vi "openSubProcess.vi"(6 "Device IDN":string, 8 "error in (no error)":errorcluster {"code" format="Error %.0f"}, 10 "notifiers":T2, 11 "messageQueues":T3) -> (0 "error out":errorcluster {"code" format="Error %.0f"}, 3 "SubViRefsOut":T1)   [LabVIEW 2017]
doc: "This VI will open and pass messageQueues and Notifier clusters to each subpanel process."
uses:
  Message Queues/messageQueues.ctl
  Message Queues/Message Cluster.ctl
  Notifiers/notifiers.ctl
  Controls/SubViRefs.ctl
  <vilib>/Utility/error.llb/Error Cluster From Error Code.vi
  <vilib>/ErrorRing/Error Ring.xnode
  Message Queues/Message Queue.lvlib
  Notifiers/notifiers.lvlib
panel:
  in  "SubViRefs":T1
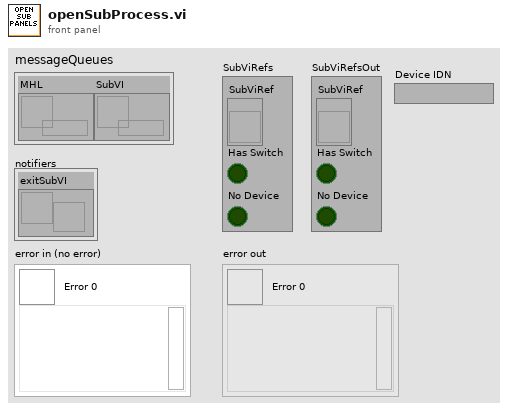
[diagram p1: front panel]
types:
  T1 = typedef "SubViRefs.ctl" = cluster{"SubViRef":refnum<vi>, "Has Switch":bool, "No Device":bool}
  T2 = typedef "notifiers.lvlib/notifiers.ctl" = cluster{"exitSubVI":refnum<notifier>}
  T3 = typedef "Message Queue.lvlib/messageQueues.ctl" = cluster{"MHL":refnum<queue>, "SubVI":refnum<queue>}
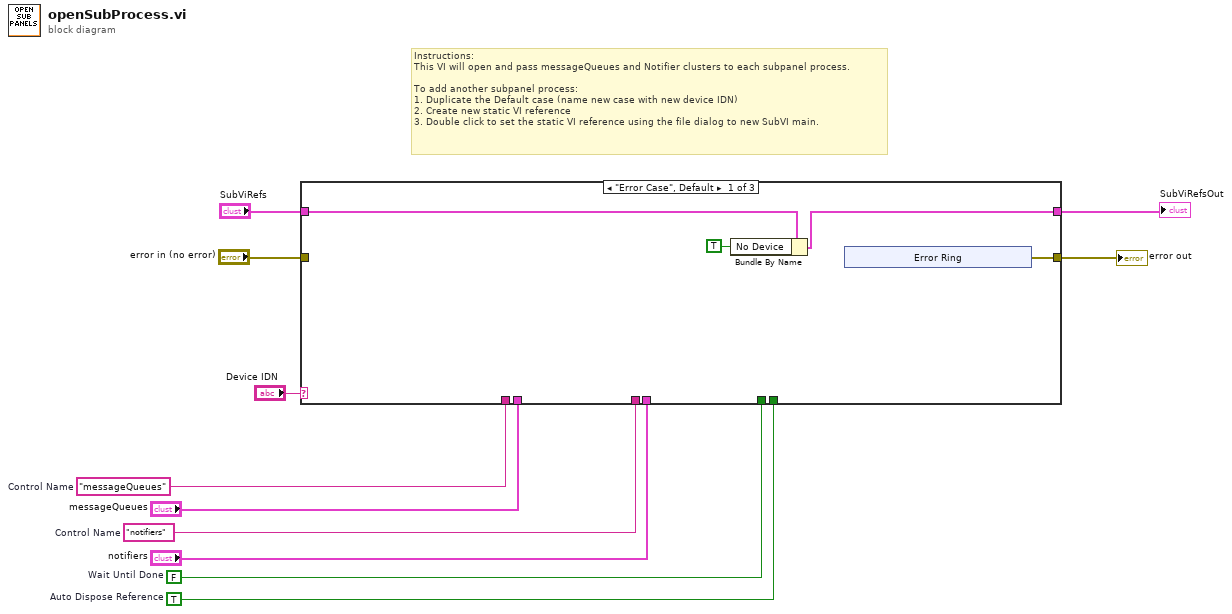
[diagram p0: block diagram]
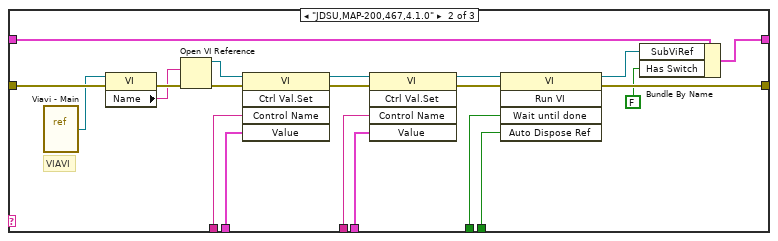
[diagram p2: hidden frame]
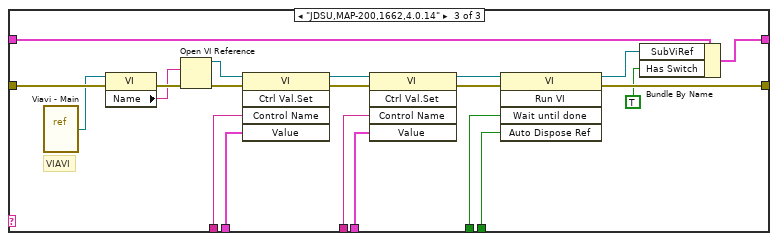
[diagram p3: hidden frame]
diagram:
  w7 = "notifiers"  # Control Name
  w4 = TRUE  # Auto Dispose Reference
  w5 = FALSE  # Wait Until Done
  w9 = "messageQueues"  # Control Name
  # "Instructions:\nThis VI will open and pass messageQueues and Notifier clusters to each subpanel process.\n\nTo add another subpanel process:\n1. Duplicate the Default case (name new case with new device IDN)\n2. Create new static VI reference\n3. Double click to set the static VI reference using the file dialog to new SubVI main."
  n1 = case shown="\"Error Case\", Default" "Device IDN" {
    tunnel: "error in (no error)" -> [_ w33 w54]
    tunnel: "SubViRefs" -> [w14 w31 w52]
    tunnel: [w13 w30 w51] -> w2
    tunnel: [w15 w29 w50] -> w10
    tunnel: w9 -> [_ w28 w49]
    tunnel: "messageQueues" -> [_ w27 w48]
    tunnel: w7 -> [_ w26 w47]
    tunnel: "notifiers" -> [_ w25 w46]
    tunnel: w5 -> [_ w24 w45]
    tunnel: w4 -> [_ w23 w44]
    frame "Error Case", Default {
      n2 = Bundle By Name(cluster=w14, "No Device"=TRUE) -> (w13:T1)
      n3 = xnode "Error Ring"() -> ("error out"=w15:errorcluster)
    }
    frame "JDSU,MAP-200,467,4.1.0" {
      # "VIAVI"
      n4 = vi-ref "Viavi - Main.vi"() -> (w22:refnum<vi>)
      n5 = property class="VI"(reference=w22, error in=w33) -> (error out=w35:errorcluster, "Name"=w34:string)  [unwired: 1 out]
      n6 = Open VI Reference(vi path=w34, error in (no error)=w35) -> (vi reference=w39:refnum<vi>, error out=w36:errorcluster)  [unwired: 4 in]
      n7 = invoke class="VI" method="Ctrl Val.Set"(reference=w39, error in=w36, "Control Name"=w28, "Value"=w27) -> (reference out=w40:refnum<vi>, error out=w38:errorcluster)  [unwired: 1 in, 3 out]
      n8 = invoke class="VI" method="Ctrl Val.Set"(reference=w40, error in=w38, "Control Name"=w26, "Value"=w25) -> (reference out=w41:refnum<vi>, error out=w37:errorcluster)  [unwired: 1 in, 3 out]
      n9 = invoke class="VI" method="Run VI"(reference=w41, error in=w37, "Wait until done"=w24, "Auto Dispose Ref"=w23) -> (reference out=w32:refnum<vi>, error out=w29:errorcluster)  [unwired: 1 in, 3 out]
      n10 = Bundle By Name(cluster=w31, "SubViRef"=w32, "Has Switch"=FALSE) -> (w30:T1)
    }
    frame "JDSU,MAP-200,1662,4.0.14" {
      # "VIAVI"
      n11 = vi-ref "Viavi - Main.vi"() -> (w43:refnum<vi>)
      n12 = property class="VI"(reference=w43, error in=w54) -> (error out=w56:errorcluster, "Name"=w55:string)  [unwired: 1 out]
      n13 = Open VI Reference(vi path=w55, error in (no error)=w56) -> (vi reference=w60:refnum<vi>, error out=w57:errorcluster)  [unwired: 4 in]
      n14 = invoke class="VI" method="Ctrl Val.Set"(reference=w60, error in=w57, "Control Name"=w49, "Value"=w48) -> (reference out=w61:refnum<vi>, error out=w59:errorcluster)  [unwired: 1 in, 3 out]
      n15 = invoke class="VI" method="Ctrl Val.Set"(reference=w61, error in=w59, "Control Name"=w47, "Value"=w46) -> (reference out=w62:refnum<vi>, error out=w58:errorcluster)  [unwired: 1 in, 3 out]
      n16 = invoke class="VI" method="Run VI"(reference=w62, error in=w58, "Wait until done"=w45, "Auto Dispose Ref"=w44) -> (reference out=w53:refnum<vi>, error out=w50:errorcluster)  [unwired: 1 in, 3 out]
      n17 = Bundle By Name(cluster=w52, "SubViRef"=w53, "Has Switch"=TRUE) -> (w51:T1)
    }
  }
  "error out" <- w10
  "SubViRefsOut" <- w2
